vi "RSNRPZ Channels Zero.vi"(8 "error in (no error)":errorcluster, 11 "VISA session":refnum<visa-resource-name> caption="VISA resource name") -> (0 "error out":errorcluster, 3 "dup VISA session":refnum<visa-resource-name> caption="VISA resource name")   [LabVIEW 2010]
doc: "This VI starts zeroing of all sensors using the signal at each sensor input. Zeroing is an asynchronous operation which will require a couple of seconds. Therefore, after starting the VI, the user should poll the current execution status by continuously calling RSNRPZ Chans Zeroing Complete State.vi. As soon as the zeroing has finished, the result of the operation can be queried by a call to RSNRPZ Error-Query.vi.\n\nNote: The sensor must be disconnected from all power sources. If the signal at the input considerably deviates from 0 W, the sensor aborts the zero calibration and raises an error condition. The rsnrpz driver queues the error for later retrieval by the RSNRPZ Error-Query.vi.\n\nbool Zero( ViSession lSesID )\n{\n const int CH1 = 1;\n ViStatus lStat = VI_SUCCESS;\n ViBoolean bZeroComplete = VI_FALSE;\n ViInt32 iErrorCode = VI_SUCCESS;\n ViChar szErrorMsg[256];\n /* Start zeroing the sensor… */\n lStat = rsnrpz_chans_zero( lSesID );\n if ( lStat != VI_SUCCESS )\n {\n fprintf( stderr, “Error 0x%08x in rsnrpz_chan_zero()\", lStat );\n return false;\n }\n while ( bZeroComplete == VI_FALSE )\n {\n lStat = rsnrpz_chans_isZeroComplete( lSesID, &bZeroComplete );\n if ( bZeroComplete )\n {\n rsnrpz_error_query( lSesID, &iErrorCode, szErrorMsg );\n fprintf( stderr, \"Zero-Cal.: error %d, %s\\n\\n\", iErrorCode, szErrorMsg );\n break;\n }\n else \n SLEEP( 200 );\n }\n return iErrorCode == 0;\n}\n\nRemote-control command(s):\nCAL:ZERO:AUTO"
uses:
  rsnrpz_32.dll
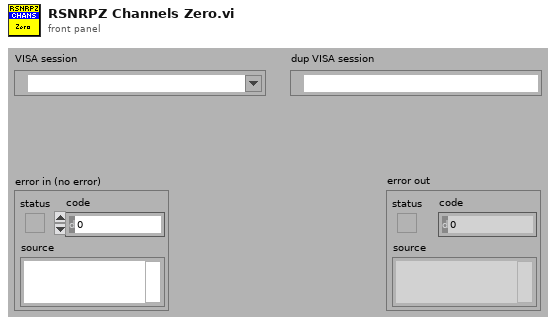
[diagram p1: front panel]
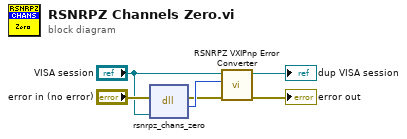
[diagram p0: block diagram]
diagram:
  n1 = dll-call lib="rsnrpz_32.dll" fn="rsnrpz_chans_zero"(error in="error in (no error)", "VISA Session"="VISA session") -> (error out=w5:errorcluster, "Status"=w6:i32)  [unwired: 3 in, 1 out]
  n2 = call <instrlib>:"RSNRPZ VXIPnp Error Converter.vi"("error in"=w5, "VXIPnp error code"=w6, "VISA session"="VISA session") -> ("error out"=→"error out":errorcluster, "dup VISA session"=→"dup VISA session":refnum<visa-resource-name>)  [unwired: 7 in]
